vi "Implement Constructor.vi"(8 "error in (no error)":errorcluster, 10 "Constructor Path":path, 11 "Mock Class Generator in":refnum<class "Mock Class Generator.lvclass">) -> (0 "error out":errorcluster, 3 "Mock Class Generator":refnum<class "Mock Class Generator.lvclass">)   [LabVIEW 2020, in "Mock Class Generator.lvclass"]
uses:
  Mock Class Generator.lvclass
  <vilib>/Utility/traverseref.llb/TRef TravTarget.ctl
  Mock Class Generator.lvclass/Mock Class Generator.ctl
  <vilib>/Utility/traverseref.llb/VI Scripting - Traverse.lvlib
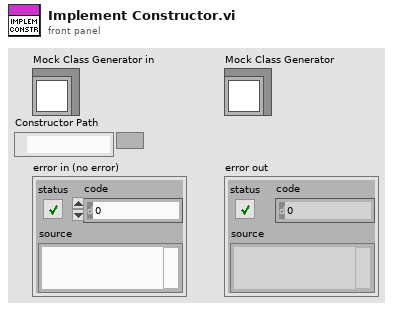
[diagram p1: front panel]
types:
  T1 = typedef "TRef TravTarget.ctl" = enum16{"FP", "BD", "Other"}
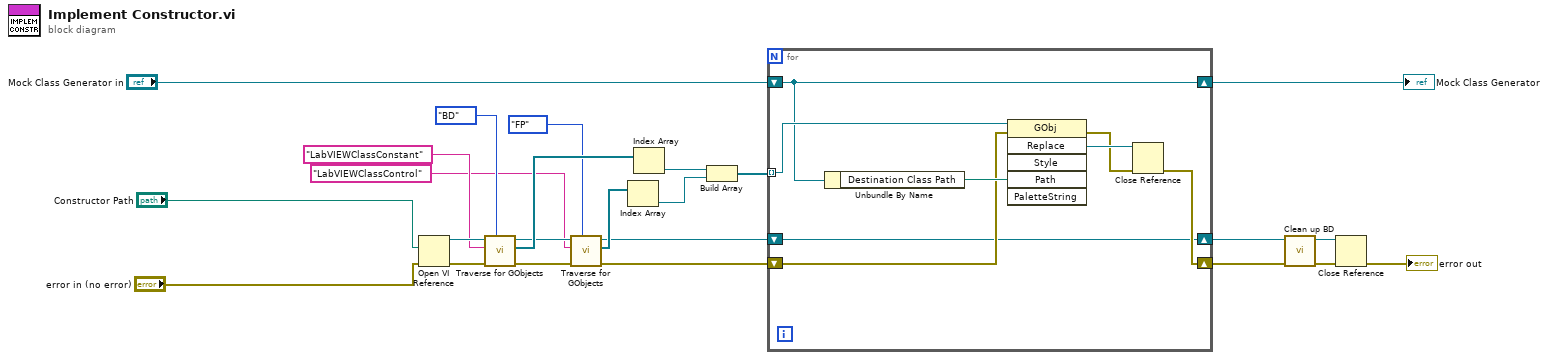
[diagram p0: block diagram]
diagram:
  n1 = Open VI Reference(vi path="Constructor Path", error in (no error)="error in (no error)") -> (vi reference=w21:refnum<vi>, error out=w24:errorcluster)  [unwired: 4 in]
  n2 = call <vilib>:"Traverse for GObjects.vi"("Traverse Target"=TRef_TravTarget."BD", "error in (no error)"=w24, "Class Name"="LabVIEWClassConstant", "VI Refnum"=w21) -> ("error out"=w12:errorcluster, "References"=w18:refnum<vi>[], "dup VI Refnum"=w13:refnum<vi>)  [unwired: 4 in, 1 out]
  n3 = call <vilib>:"Traverse for GObjects.vi"("Traverse Target"=TRef_TravTarget."FP", "error in (no error)"=w12, "Class Name"="LabVIEWClassControl", "VI Refnum"=w13) -> ("error out"=w3:errorcluster, "References"=w9:refnum<vi>[], "dup VI Refnum"=w2:refnum<vi>)  [unwired: 4 in, 1 out]
  n4 = Index Array(array=w9) -> (element=w8:refnum<vi>)  [unwired: 1 in]
  n5 = Index Array(array=w18) -> (element=w17:refnum<vi>)  [unwired: 1 in]
  n6 = Build Array(w17, w8) -> (w15:refnum<vi>[])
  n7 = for {
    tunnel: w15 -> [w31] mode=indexing
    shift-right: [w26] -> w5
    shift-left: w3 -> [w30]
    shift-right: [w28] -> w14
    shift-left: "Mock Class Generator in" -> [w28]
    shift-right: [w25] -> w1
    shift-left: w2 -> [w25]
    n8 = Unbundle By Name(w28) -> ("Destination Class Path"=w32:path)
    n9 = invoke class="GObj" method="Replace"(reference=w31, error in=w30, "Path"=w32) -> (error out=w27:errorcluster, "Replace"=w29:refnum<vi>)  [unwired: 3 in, 4 out]
    n10 = Close Reference(reference=w29, error in (no error)=w27) -> (error out=w26:errorcluster)
  }
  "Mock Class Generator" <- w14
  n11 = call "Clean up BD.vi"("error in (no error)"=w5, "VI in"=w1) -> ("error out"=w7:errorcluster, "VI out"=w6:refnum<vi>)  [unwired: 8 in]
  n12 = Close Reference(reference=w6, error in (no error)=w7) -> (error out=→"error out":errorcluster)
